vi "show_history.vi"(8 "error in (no error)":errorcluster, 11 "HR Data Structure":T1={"Runer's Data"={"Name"="", "Age"=0}, "HR Max"=0, "Raw Data"={"Time"=[], "Bpm"=[]}, "% HR MAX "=[], "HR Zones "=[], "no of points"=[], "Heart Rate Zone No 2"=[1, 2, 3, 4, 5], "History"=[["training number", "HR Max value", "HR Mean value"], ["", "", ""]], "number history"=0}) -> (0 "error in (no error) 2":errorcluster)   [LabVIEW 2024]
uses:
  zad_3-labview/klaster 4.ctl
  zad_3-labview/klaster.ctl
  zad_3-labview/klaster 2.ctl
panel:
  out "Historia treningów":string[][](array[string])
  in  "Button":bool
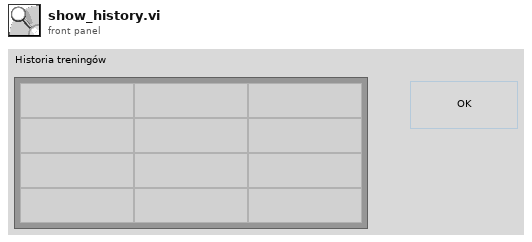
[diagram p1: front panel]
types:
  T1 = typedef "klaster 4.ctl" = cluster{"Runer's Data":T2, "HR Max":i32, "Raw Data":T3, "% HR MAX ":dbl[], "HR Zones ":string[][], "no of points":dbl[], "Heart Rate Zone No 2":i32[], "History":string[][], "number history":i32}
  T2 = typedef "klaster.ctl" = cluster{"Name":string, "Age":i32}
  T3 = typedef "klaster 2.ctl" = cluster{"Time":timestamp[], "Bpm":i32[]}
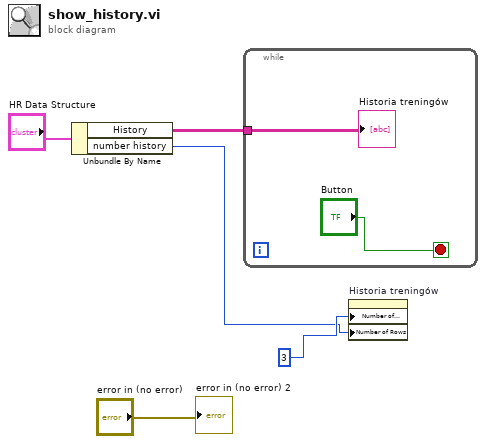
[diagram p0: block diagram]
diagram:
  n1 = Unbundle By Name("HR Data Structure") -> ("History"=w4:string[][], "number history"=w2:i32)
  n2 = while {
    tunnel: w4 -> [w6]
    stop <- "Button" stop-if-true
    "Historia treningów" <- w6
  }
  n3 = property on="Historia treningów" class="Arr (strict)"("Number of Columns"=u32 3, "Number of Rows"=w2) -> ()  [unwired: 2 in, 2 out]
  "error in (no error) 2" <- "error in (no error)"
